vi "Encoder Loop.vi"() -> (3 "Encoder Data":T1 {"Omni"."Ticks" format="%#.6g"; "Right"."Ticks" format="%#.6g"; "Left"."Ticks" format="%#.6g"})   [LabVIEW 2013]
uses:
  Sensors/Encoder Data.ctl
  Sensors/Single Encoder Data.ctl
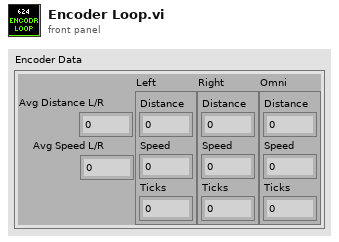
[diagram p1: front panel]
types:
  T1 = typedef "Encoder Data.ctl" = cluster{"Avg Distance L/R":dbl, "Avg Speed L/R":dbl, "Left":T2, "Right":T2, "Omni":T2}
  T2 = typedef "Single Encoder Data.ctl" = cluster{"Distance":dbl, "Speed":dbl, "Ticks":dbl}
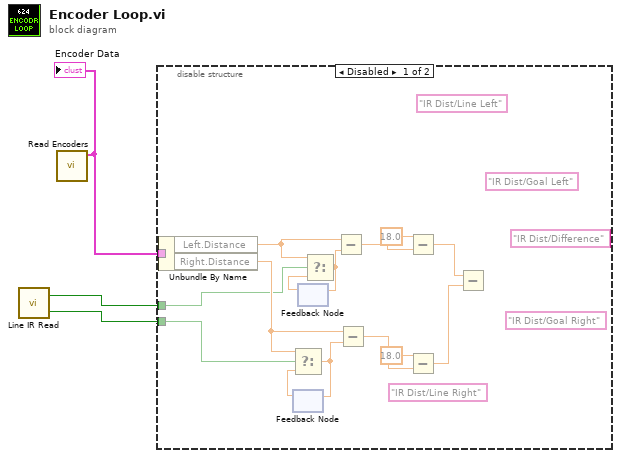
[diagram p0: block diagram]
diagram:
  n1 = call "Line IR Read.vi"() -> ("Line IR Right"=w1:bool, "Line IR Left"=w3:bool)  [unwired: 2 in]
  n2 = call "Read Encoders.vi"() -> ("Encoder Data"=w2:T1)  [unwired: 11 in]
  "Encoder Data" <- w2
  n3 = disable-structure shown="Disabled" {
    disable-tunnel: w3 -> [w6 _]
    disable-tunnel: w2 -> [w5 _]
    disable-tunnel: w1 -> [w4 _]
    frame Disabled {
      (unwired) "IR Dist/Difference" ("Name")
      w23 = "IR Dist/Goal Right" ("Name")
      w22 = "IR Dist/Goal Left" ("Name")
      w21 = "IR Dist/Line Right" ("Name")
      w20 = "IR Dist/Line Left" ("Name")
      n4 = Unbundle By Name(w5) -> ("Left.Distance"=w9:dbl, "Right.Distance"=w10:dbl)
      n5 = feedback #1() -> (w13:dbl)  [unwired: 1 in]
      n6 = Select(t=w10, s=w4, f=w13) -> (s? t:f=w12:dbl)
      n7 = feedback-in #1(w12) -> ()
      n8 = feedback #2() -> (w8:dbl)  [unwired: 1 in]
      n9 = Select(t=w9, s=w6, f=w8) -> (s? t:f=w7:dbl)
      n10 = feedback-in #2(w7) -> ()
      n11 = Subtract(x=w9, y=w7) -> (x-y=w17:dbl)
      n12 = Subtract(x=w10, y=w12) -> (x-y=w11:dbl)
      n13 = Subtract(x=18.0 ("abs(x)"), y=w17) -> (x-y=w16:dbl)
      n14 = Subtract(x=18.0, y=w11) -> (x-y=w14:dbl)
      n15 = Subtract(x=w16, y=w14) -> (x-y=w15:dbl)
    }
    frame Enabled {
    }
  }
